vi "Out_Off_N4_X01.vi"(4 "Driver Name":T10, 6 "Error Code":T11, 7 "SwitchOFF":T7=TRUE, 8 "error in":T9, 11 "DriverConnect in":T1={"InterfaceType"=enum."VISA", "OpenedSession"="", "InterfaceSettings"={"Interface"=enum."RS232", "EOS 4 read"=enum."LF (\\n)", "EOS 4 write"=enum."LF (\\n)", "TMO, ms"=10000, "Sett"=variant(cluster{"Baud Rate":u32, "Data Bits":u16, "Parity":u16, "Stop Bits":u16, "Flow Control":u16, "Eho":bool} {"Baud Rate"=75, "Data Bits"=0, "Parity"=0, "Stop Bits"=0, "Flow Control"=0, "Eho"=FALSE})}}) -> (0 "error out":T9, 3 "DriverConnect out":T1={"InterfaceType"=enum."VISA", "OpenedSession"="", "InterfaceSettings"={"Interface"=enum."RS232", "EOS 4 read"=enum."LF (\\n)", "EOS 4 write"=enum."LF (\\n)", "TMO, ms"=10000, "Sett"=variant(cluster{"Baud Rate":u32, "Data Bits":u16, "Parity":u16, "Stop Bits":u16, "Flow Control":u16, "Eho":bool} {"Baud Rate"=75, "Data Bits"=0, "Parity"=0, "Stop Bits"=0, "Flow Control"=0, "Eho"=FALSE})}})   [LabVIEW 2018]
uses:
  MOKO_LabViewLibrary/MokoLowLevel/MokoLowLovelControl/MLLC_ErrorCode.ctl
  MOKO_LabViewLibrary/MokoLowLevel/MokoLowLovelControl/MLLC_DriverName.ctl
  MOKO_LabViewLibrary/MokoLowLevel/MokoLowLovelControl/MLLC_Error.ctl
  MOKO_LabViewLibrary/MokoLowLevel/MokoLowLovelControl/MLLC_Delay.ctl
  MOKO_LabViewLibrary/MokoLowLevel/MokoLowLovelControl/MLLC_Boolean.ctl
  MOKO_LabViewLibrary/MokoLowLevel/MokoLowLovelControl/MLLC_Command.ctl
  MOKO_LabViewLibrary/MokoLowLevel/MokoLowLovelControl/MLLC_ConnectCluster.ctl
  MOKO_LabViewLibrary/MokoLowLevel/MokoLowLovelControl/MLLC_InterfaceType.ctl
  MOKO_LabViewLibrary/MokoLowLevel/MokoLowLovelControl/MLLC_OpenedSession.ctl
  MOKO_LabViewLibrary/MokoLowLevel/MokoLowLovelControl/MLLC_InterfaceSettings.ctl
  MOKO_LabViewLibrary/MokoLowLevel/MokoLowLovelControl/MLLC_InterfaceKind.ctl
panel:
  out "Array":T6[](array[typedef])
  out "iterations":T8
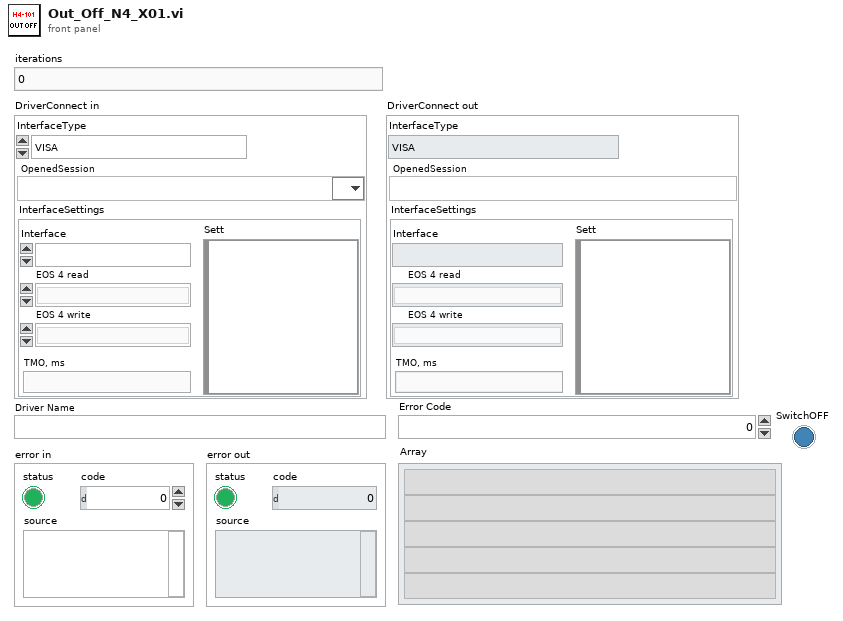
[diagram p1: front panel]
types:
  T1 = typedef "MLLC_ConnectCluster.ctl" = cluster{"InterfaceType":T2, "OpenedSession":T3, "InterfaceSettings":T4}
  T2 = typedef "MLLC_InterfaceType.ctl" = enum16{"VISA", "Prologix USB-GPIB"}
  T3 = typedef "MLLC_OpenedSession.ctl" = refnum<visa-resource-name>
  T4 = typedef "MLLC_InterfaceSettings.ctl" = cluster{"Interface":T5, "EOS 4 read":enum16{"Default (=EOS 4 write)", "CR (\\r)", "LF (\\n)", "None"}, "EOS 4 write":enum16{"CR+LF (\\r\\n)", "CR (\\r)", "LF (\\n)", "None"}, "TMO, ms":i32, "Sett":variant}
  T5 = typedef "MLLC_InterfaceKind.ctl" = enum16{"RS232", "GPIB", "USB", "Ethernet", "another"}
  T6 = typedef "MLLC_Command.ctl" = string
  T7 = typedef "MLLC_Boolean.ctl" = bool
  T8 = typedef "MLLC_Delay.ctl" = dbl
  T9 = typedef "MLLC_Error.ctl" = errorcluster
  T10 = typedef "MLLC_DriverName.ctl" = string
  T11 = typedef "MLLC_ErrorCode.ctl" = u32
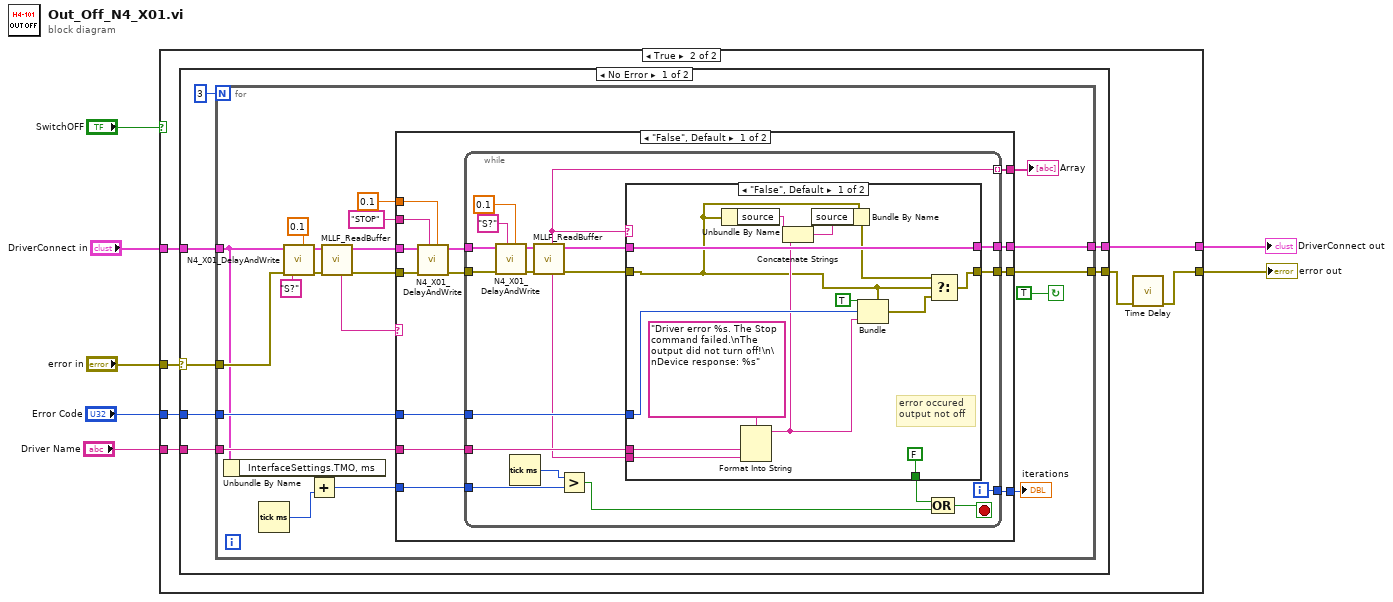
[diagram p0: block diagram]
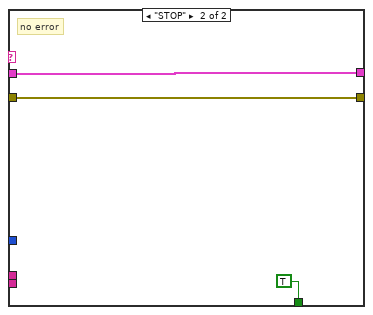
[diagram p3: hidden frame]
diagram:
  n1 = case shown="True" "SwitchOFF" {
    tunnel: [w8 w11] -> w3
    tunnel: [w9 w16] -> w1
    tunnel: "Error Code" -> [_ w15]
    tunnel: "Driver Name" -> [_ w14]
    tunnel: "DriverConnect in" -> [w9 w13]
    tunnel: "error in" -> [w8 w12]
    frame False {
    }
    frame True {
      n2 = case shown="No Error" w12 {
        selector: w12 -> [w18 w97]
        tunnel: [w23 w97] -> w10
        tunnel: [w22 w96] -> w16
        tunnel: w15 -> [w21 _]
        tunnel: w14 -> [w20 _]
        tunnel: w13 -> [w19 w96]
        frame No Error {
          n3 = for {
            N: 3 -> [_]
            tunnel: [w26] -> w23
            tunnel: [w44] -> w22
            tunnel: w21 -> [w43]
            tunnel: w20 -> [w42]
            tunnel: w19 -> [w24]
            tunnel: w18 -> [w35]
            stop <- TRUE continue-if-true
            n4 = Unbundle By Name(w24) -> ("InterfaceSettings.TMO, ms"=w40:i32)
            n5 = Tick Count (ms)() -> (millisecond timer value=w41:u32)
            n6 = call "N4_X01_DelayAndWrite.vi"("Delay Befor (s)"=0.1, "Command"="S?" ("Error Query"), "error in"=w35, "DriverConnect in"=w24) -> ("error out"=w33:T9, "DriverConnect out"=w32:T1)  [unwired: 6 in]
            n7 = Add(x=w40, y=w41) -> (x+y=w39:u32)
            n8 = call "MLLF_ReadBuffer.vi"("Error In"=w33, "DriverConnect in"=w32) -> ("Error Out"=w30:errorcluster, "DriverConnect out"=w31:T1, "String"=w29:string)  [unwired: 6 in]
            n9 = case shown="\"False\", Default" w29 {
              tunnel: [w57 w95] -> w26
              tunnel: [w56 w94] -> w44
              tunnel: w43 -> [w55 _]
              tunnel: w42 -> [w54 _]
              tunnel: w39 -> [w53 _]
              tunnel: [w52 _] -> w38
              tunnel: [w51 _] -> w27
              tunnel: "STOP" ("String") -> [w50 _]
              tunnel: 0.1 ("Delay Befor (s)") -> [w49 _]
              tunnel: w31 -> [w46 w94]
              tunnel: w30 -> [w45 w95]
              frame "False", Default {
                n10 = call "N4_X01_DelayAndWrite.vi"("Delay Befor (s)"=w49, "Command"=w50, "error in"=w45, "DriverConnect in"=w46) -> ("error out"=w47:T9, "DriverConnect out"=w48:T1)  [unwired: 6 in]
                n11 = while {
                  tunnel: w48 -> [w59]
                  tunnel: w47 -> [w58]
                  tunnel: [w72] -> w57
                  tunnel: [w71] -> w56
                  tunnel: w55 -> [w70]
                  tunnel: w54 -> [w69]
                  tunnel: w53 -> [w67]
                  tunnel: [w63] -> w52
                  tunnel: [w60] -> w51 mode=indexing
                  i -> [w63]
                  stop <- w66 stop-if-true
                  n12 = call "N4_X01_DelayAndWrite.vi"("Delay Befor (s)"=0.1, "Command"="S?" ("Error Query"), "error in"=w58, "DriverConnect in"=w59) -> ("error out"=w62:T9, "DriverConnect out"=w76:T1)  [unwired: 6 in]
                  n13 = Tick Count (ms)() -> (millisecond timer value=w68:u32)
                  n14 = call "MLLF_ReadBuffer.vi"("Error In"=w62, "DriverConnect in"=w76) -> ("Error Out"=w73:errorcluster, "DriverConnect out"=w74:T1, "String"=w60:string)  [unwired: 6 in]
                  n15 = Greater?(x=w68, y=w67) -> (0:w64:bool)
                  n16 = case shown="\"False\", Default" w60 {
                    tunnel: w74 -> [w90 w92]
                    tunnel: w73 -> [w77 w93]
                    tunnel: [w79 w93] -> w72
                    tunnel: [w90 w92] -> w71
                    tunnel: w70 -> [w87 _]
                    tunnel: w69 -> [w86 _]
                    tunnel: [FALSE TRUE] -> w65
                    tunnel: w60 -> [w80 _]
                    frame "False", Default {
                      # "error occured\noutput not off"
                      n17 = Unbundle By Name(w77) -> ("source"=w83:string)
                      n18 = Format Into String(format string="Driver error %s. The Stop command failed.\nThe output did not turn off!\n\nDevice response: %s", w86, w80) -> (resulting string=w82:string)  [unwired: 2 in, 1 out]
                      n19 = Concatenate Strings(w83, w82) -> (w84:string)
                      n20 = Bundle By Name(cluster=w77, "source"=w84) -> (w81:errorcluster)
                      n21 = Bundle(cluster=w77, "status"=TRUE ("Status"), "code"=w87, "source"=w82) -> (w78:errorcluster)
                      n22 = Select(t=w81, s=w77, f=w78) -> (s? t:f=w79:errorcluster)
                    }
                    frame "STOP" {
                      # "no error"
                    }
                  }
                  n23 = Compound Arithmetic op=OR(w65, w64) -> (w66:bool)
                }
              }
              frame "stop" {
              }
            }
            "iterations" <- w38
            "Array" <- w27
          }
        }
        frame Error {
        }
      }
      n24 = call "Time Delay"("error in (no error)"=w10) -> ("error out"=w11:errorcluster)  [unwired: 10 in]
    }
  }
  "error out" <- w3
  "DriverConnect out" <- w1
